vi "GetThermocoupleProperties.vi"(11 "Properties":T1[](array[typedef])) -> (2 "AI Thermocouple type":u32, 3 "AI degree range":u32)   [LabVIEW 2017, in "ScanEngine.lvlib"]
uses:
  <vilib>/addons/InsightCM/Devices/Shared/Common/ScanEngine/ScanEngine.lvlib
  <vilib>/addons/InsightCM/MessageBus/Base/controls/KeyValuePair.ctl
  <vilib>/addons/InsightCM/Utilities/PropertyHelpers/PropertyHelpers.lvlib
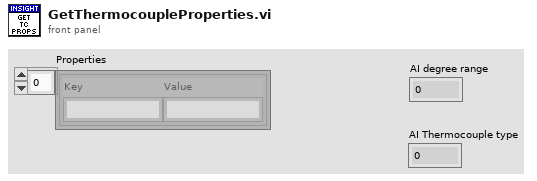
[diagram p1: front panel]
types:
  T1 = typedef "KeyValuePair.ctl" = cluster{"Key":string, "Value":string}
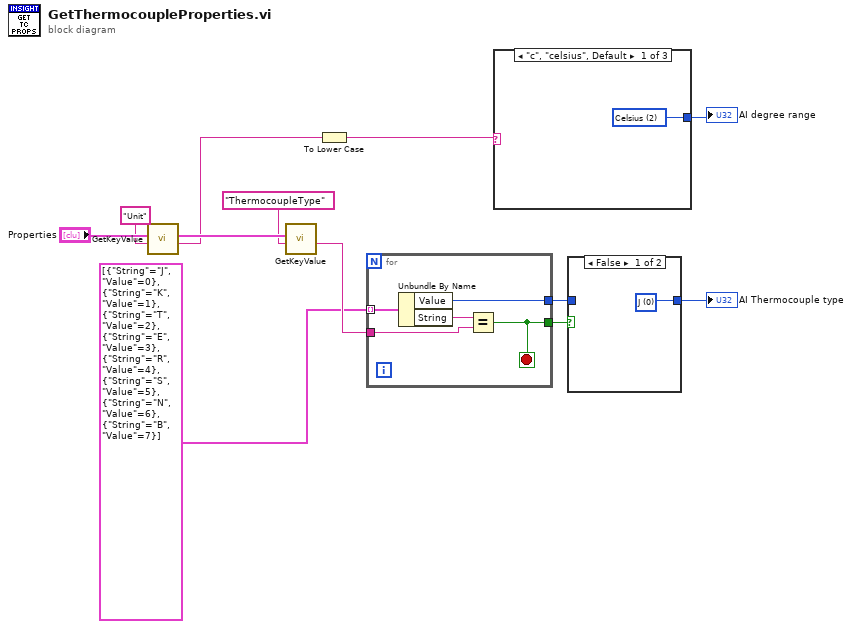
[diagram p0: block diagram]
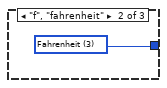
[diagram p2: hidden frame]
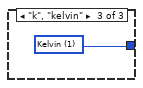
[diagram p3: hidden frame]
diagram:
  n1 = call <vilib>:"GetKeyValue.vi"("key"="Unit" ("name"), "key value pairs"="Properties") -> ("value"=w3:string, "key value pairs out"=w8:T1[])  [unwired: 7 in, 1 out]
  n2 = call <vilib>:"GetKeyValue.vi"("key"="ThermocoupleType" ("name"), "key value pairs"=w8) -> ("value"=w5:string)  [unwired: 7 in, 2 out]
  n3 = To Lower Case(string=w3) -> (all lower case string=w2:string)
  n4 = for {
    tunnel: [w16] -> w12
    tunnel: w5 -> [w15]
    tunnel: [w14] -> w11
    tunnel: cluster{"String":string, "Value":u32}[] [{"String"="J", "Value"=0}, {"String"="K", "Value"=1}, {"String"="T", "Value"=2}, {"String"="E", "Value"=3}, {"String"="R", "Value"=4}, {"String"="S", "Value"=5}, {"String"="N", "Value"=6}, {"String"="B", "Value"=7}] ("Strings And Values []") -> [w13] mode=indexing
    stop <- w14 stop-if-true
    n5 = Unbundle By Name(w13) -> ("Value"=w16:u32, "String"=w17:string)
    n6 = Equal?(x=w17, y=w15) -> (x = y?=w14:bool)
  }
  n7 = case shown="\"c\", \"celsius\", Default" w2 {
    tunnel: [w18 w19 w20] -> w4
    frame "c", "celsius", Default {
      w18 = u32 2 items=["Ohms", "Kelvin", "Celsius", "Fahrenheit", "Rankine"] ("RTD0:Ohm degree range")
    }
    frame "f", "fahrenheit" {
      w19 = u32 3 items=["Volts", "Kelvin", "Celsius", "Fahrenheit", "Rankine"] ("CH3:Degree range")
    }
    frame "k", "kelvin" {
      w20 = u32 1 items=["Volts", "Kelvin", "Celsius", "Fahrenheit", "Rankine"] ("CH3:Degree range")
    }
  }
  "AI degree range" <- w4
  n8 = case shown="False" w11 {
    tunnel: [w21 w22] -> w10
    tunnel: w12 -> [_ w22]
    frame False {
      w21 = u32 0 items=["J", "K", "T", "E", "R", "S", "N", "B"] ("AI0:Thermocouple type")
    }
    frame True {
    }
  }
  "AI Thermocouple type" <- w10
